vi "set_outputs.vi"(11 "Outputs":T1) -> ()   [LabVIEW 2012]
uses:
  Outputs.ctl
  mecanum/mecanum_output.ctl
  Shooter/shooter_outputs.ctl
  climber/climber_outputs.ctl
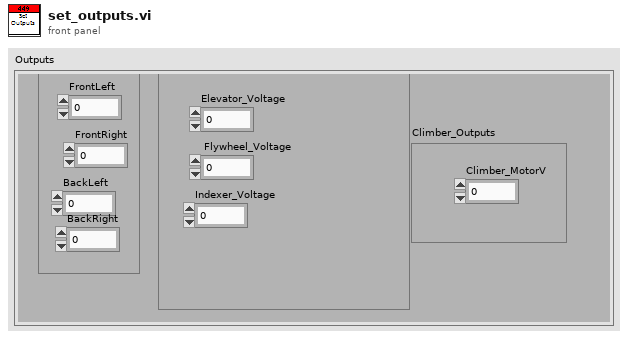
[diagram p1: front panel]
types:
  T1 = typedef "Outputs.ctl" = cluster{"Mecanum":T2, "Shooter_Outputs":T3, "Climber_Outputs":T4}
  T2 = typedef "mecanum_output.ctl" = cluster{"FrontLeft":dbl, "FrontRight":dbl, "BackLeft":dbl, "BackRight":dbl}
  T3 = typedef "shooter_outputs.ctl" = cluster{"Elevator_Voltage":dbl, " Flywheel_Voltage":dbl, "Indexer_Voltage":dbl}
  T4 = typedef "climber_outputs.ctl" = cluster{"Climber_MotorV":dbl}
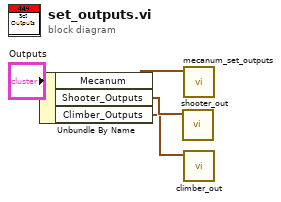
[diagram p0: block diagram]
diagram:
  n1 = Unbundle By Name("Outputs") -> ("Mecanum"=w3:T2, "Shooter_Outputs"=w2:T3, "Climber_Outputs"=w1:T4)
  n2 = call "shooter_out.vi"("Shooter_Outputs"=w2) -> ()  [unwired: 11 in]
  n3 = call "mecanum_set_outputs.vi"("Mecanum"=w3) -> ()  [unwired: 11 in]
  n4 = call "climber_out.vi"("Climber_Outputs"=w1) -> ()  [unwired: 11 in]
